vi "Proxy_GetData.vi"(8 "error in (no error)":errorcluster, 11 "VISA resource name":refnum<visa-resource-name>) -> (0 "error out":errorcluster, 1 "Read String":string, 2 "Time":timestamp, 3 "VISA resource name out":refnum<visa-resource-name>)   [LabVIEW 2019]
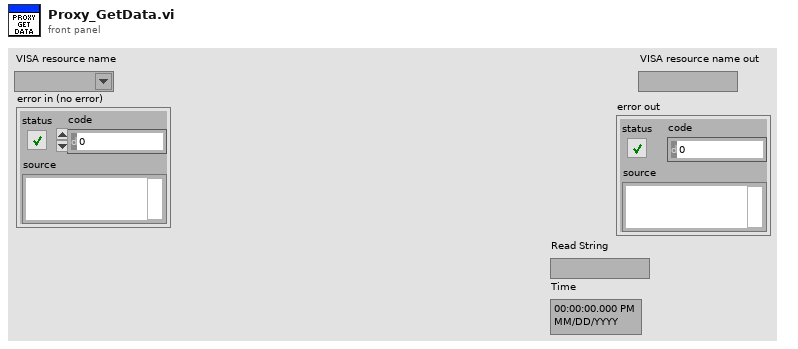
[diagram p1: front panel]
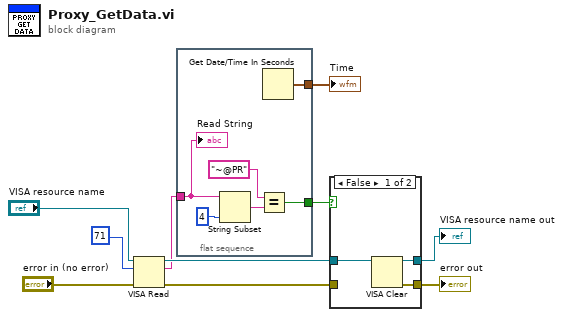
[diagram p0: block diagram]
diagram:
  n1 = VISA Read(VISA resource name="VISA resource name", byte count=u32 71, error in (no error)="error in (no error)") -> (VISA resource name out=w9:refnum<visa-resource-name>, read buffer=w4:string, error out=w7:errorcluster)  [unwired: 1 out]
  n2 = flat-sequence {
    tunnel: [w13] -> w10
    tunnel: w4 -> [w12]
    tunnel: [w11] -> w3
    frame #0 {
      n3 = String Subset(string=w12, length (rest)=4 ("length (rest)")) -> (substring=w14:string)  [unwired: 1 in]
      n4 = Equal?(x="~@PR", y=w14) -> (x = y?=w13:bool)
      n5 = Get Date/Time In Seconds() -> (seconds since 1Jan1904=w11:timestamp)
      "Read String" <- w12
    }
  }
  n6 = case shown="False" w10 {
    tunnel: w9 -> [w19 w21]
    tunnel: [w18 w21] -> w8
    tunnel: w7 -> [_ w20]
    tunnel: [w17 w20] -> w6
    frame False {
      n7 = VISA Clear(VISA resource name=w19) -> (VISA resource name out=w18:refnum<visa-resource-name>, error out=w17:errorcluster)  [unwired: 1 in]
    }
    frame True {
    }
  }
  "VISA resource name out" <- w8
  "error out" <- w6
  "Time" <- w3
